vi "CANopenWriteSDO.vi"(4 "data array":u8[](array[numeric])=[0, 0, 0, 0] format="%.0x", 6 "Byte0 (h40)":u8=64 format="%.0x", 7 "Node ID":u32=1, 8 "error in":errorcluster, 9 "Sub Index":u8 format="%.0x", 10 "Index":u16 format="%.0x", 11 "FPGA VI Reference In":refnum<k20>) -> (0 "error out":errorcluster, 3 "FPGA VI Reference Out":refnum<k20>)   [LabVIEW 2016]
doc: "This VI writes a SDO Request message to a particular node. It writes directly to the Bus, because it is not periodic."
uses:
  <vilib>/Utility/error.llb/Error Cluster From Error Code.vi
  <vilib>/rvi/errors/niLvFpgaAdjustHostInterfaceError.vi
  <vilib>/rvi/interface/nirviReadWriteControl/nirviReadWriteControl.xnode
  FPGA Bitfiles/EV-MCU_FPGATarget_CANEngine(FPGA)b_eM8Xz3qYJVA.lvbitx
  CAN_Engine(FPGA)_basic.vi
  NiFpgaLv.dll
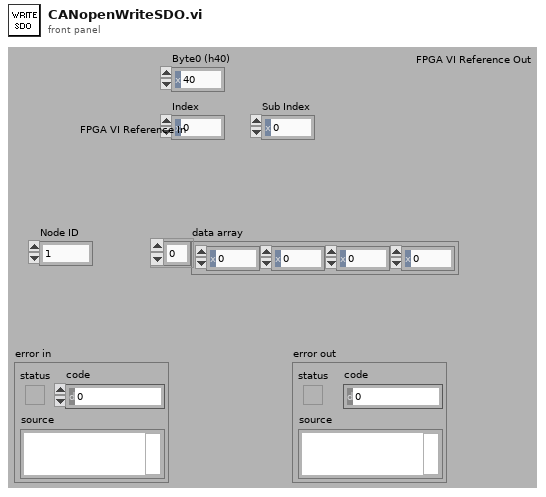
[diagram p1: front panel]
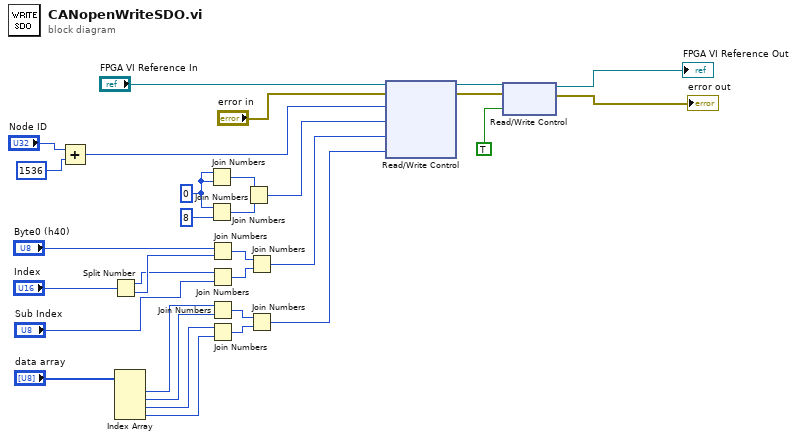
[diagram p0: block diagram]
diagram:
  w22 = u8 0 ("lo")
  n1 = Add(x="Node ID", y=u32 1536) -> (x+y=w23:u32)
  n2 = Split Number(x="Index") -> (hi(x)=w11:u8, lo(x)=w12:u8)
  n3 = Index Array(array="data array") -> (element #1=w8:u8, element #2=w7:u8, element #3=w6:u8, element #4=w5:u8)  [unwired: 4 in]
  n4 = Join Numbers(hi=w22, lo=w22) -> ((hi.lo)=w20:u16)
  n5 = Join Numbers(hi=w22, lo=u8 8 ("DataLength")) -> ((hi.lo)=w19:u16)
  n6 = Join Numbers(hi="Byte0 (h40)", lo=w12) -> ((hi.lo)=w17:u16)
  n7 = Join Numbers(hi=w11, lo="Sub Index") -> ((hi.lo)=w14:u16)
  n8 = Join Numbers(hi=w8, lo=w7) -> ((hi.lo)=w16:u16)
  n9 = Join Numbers(hi=w6, lo=w5) -> ((hi.lo)=w15:u16)
  n10 = Join Numbers(hi=w20, lo=w19) -> ((hi.lo)=w18:u32)
  n11 = Join Numbers(hi=w17, lo=w14) -> ((hi.lo)=w4:u32)
  n12 = Join Numbers(hi=w16, lo=w15) -> ((hi.lo)=w3:u32)
  n13 = xnode "Read/Write Control"("FPGA VI Reference In"="FPGA VI Reference In", "error in"="error in", "U32 Out 3"=w23, "U32 Out 4"=w18, "U32 Out 5"=w4, "U32 Out 6"=w3) -> ("FPGA VI Reference Out"=w30:refnum<k20>, "error out"=w29:errorcluster)
  n14 = xnode "Read/Write Control"("FPGA VI Reference In"=w30, "error in"=w29, "Write"=TRUE ("New Transmit")) -> ("FPGA VI Reference Out"=→"FPGA VI Reference Out":refnum<k20>, "error out"=→"error out":errorcluster)
